vi "ADC.vi"() -> ()   [LabVIEW 2010]
panel:
  in  "ADC Rate":i32
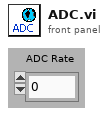
[diagram p1: front panel]
diagram:
